vi "RichToFlathwval_EmptyRequest.vi"(5 "OutputClusterType":T1, 11 "InputCluster":T2) -> (3 "OutputCluster":T1)   [LabVIEW 2025, in "ExamplePluginOOBService_server.lvlib"]
uses:
  ExamplePluginOOBService_server.lvlib
  hwval_EmptyRequest.ctl
  hwval_EmptyRequest_Flat.ctl
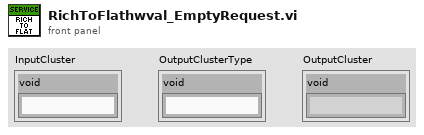
[diagram p1: front panel]
types:
  T1 = typedef "ExamplePluginOOBService_server.lvlib/hwval_EmptyRequest_Flat.ctl" = cluster{"void":string}
  T2 = typedef "ExamplePluginOOBService_server.lvlib/hwval_EmptyRequest.ctl" = cluster{"void":string}
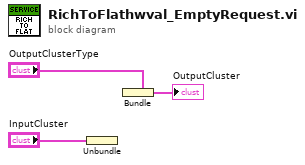
[diagram p0: block diagram]
diagram:
  n1 = Unbundle "Unbundle"("InputCluster") -> ()  [unwired: 1 out]
  n2 = Bundle "Bundle"(cluster="OutputClusterType") -> (→"OutputCluster":T1)  [unwired: 1 in]
